vi "Write Waveforms_no format path.vi"(7 "Application Directory":path, 11 "Semiconductor Module Context":T1) -> (0 "error out":errorcluster)   [LabVIEW 2013]
uses:
  <vilib>/NI_TestStand_SemiconductorModule/NI_TestStand_Semiconductor_Module.lvlibp/PinMap/General/SemiconductorModuleContext.ctl
  <instrlib>/niHSDIO/niHSDIO.llb/niHSDIO Write Named Waveform From File (HWS).vi
  <vilib>/NI_TestStand_SemiconductorModule/NI_TestStand_Semiconductor_Module.lvlibp
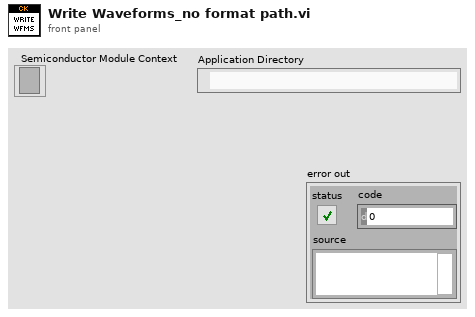
[diagram p1: front panel]
types:
  T1 = typedef "NI_TestStand_Semiconductor_Module.lvlibp/SemiconductorModuleContext.ctl" = refnum<k7>
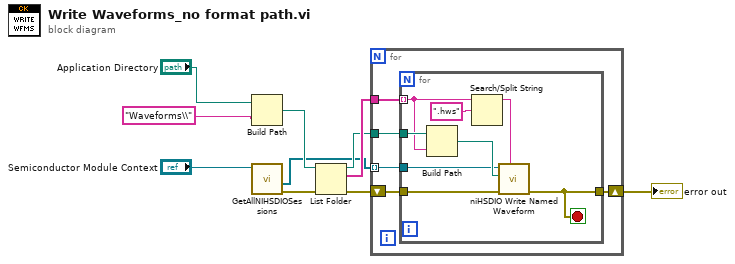
[diagram p0: block diagram]
diagram:
  n1 = Build Path(base path="Application Directory", name or relative path="Waveforms\\" ("string")) -> (appended path=w6:path)
  n2 = call <vilib>:"GetAllNIHSDIOSessions.vi"("Semiconductor Module Context"="Semiconductor Module Context") -> ("error out"=w3:errorcluster, "Generation Sessions"=w5:refnum<k15>[])  [unwired: 7 in, 2 out]
  n3 = List Folder(path=w6, error in=w3) -> (path out=w7:path, filenames=w8:string[], error out=w2:errorcluster)  [unwired: 2 in, 1 out]
  n4 = for {
    tunnel: w8 -> [w15]
    tunnel: w7 -> [w14]
    tunnel: w5 -> [w13] mode=indexing
    shift-right: [w11] -> w4
    shift-left: w2 -> [w12]
    n5 = for {
      tunnel: w15 -> [w21] mode=indexing
      tunnel: w14 -> [w22]
      tunnel: w13 -> [w18]
      tunnel: w12 -> [w17]
      tunnel: [w16] -> w11
      stop <- w16 stop-if-true
      n6 = Build Path(base path=w22, name or relative path=w21) -> (appended path=w19:path)
      n7 = Search/Split String(string=w21, search string/char (-)=".hws") -> (substring before match=w20:string)  [unwired: 1 in, 2 out]
      n8 = call-poly <instrlib>:"niHSDIO Write Named Waveform.vi"("waveform name (default:\"\")"=w20, "error in (no error)"=w17, "file path"=w19, "instrument handle"=w18) -> ("error out"=w16:errorcluster)  [unwired: 5 in, 2 out]
    }
  }
  "error out" <- w4
